vi "Read Open Thermocouple Detection.vi"(8 "error in":errorcluster, 11 "NI 9212 in":refnum<class "NI 9212.lvclass">) -> (0 "error out":errorcluster, 2 "open thermocouple detection":bool, 3 "NI 9212 out":refnum<class "NI 9212.lvclass">)   [LabVIEW 2020, in "Scan Engine Scripting.lvlib" / "NI 9212.lvclass"]
uses:
  NI 9212.lvclass
  NI 9212.lvclass/NI 9212.ctl
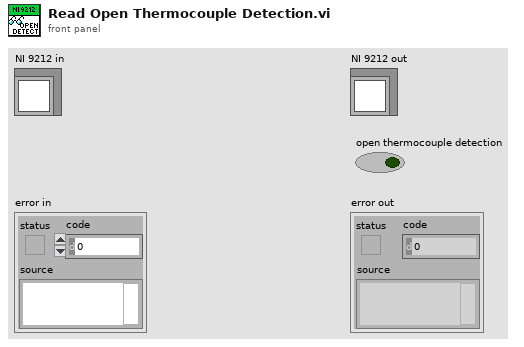
[diagram p1: front panel]
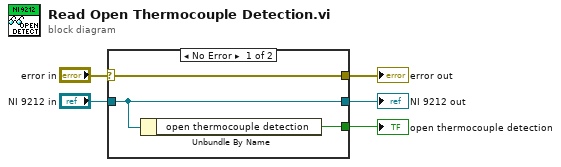
[diagram p0: block diagram]
diagram:
  n1 = case shown="No Error" "error in" {
    selector: "error in" -> [w8 w9]
    tunnel: [w8 w9] -> w4
    tunnel: [w7 w10] -> w2
    tunnel: "NI 9212 in" -> [w7 w10]
    tunnel: [w6 _] -> w1
    frame No Error {
      n2 = Unbundle By Name(w7) -> ("open thermocouple detection"=w6:bool)
    }
    frame Error {
    }
  }
  "error out" <- w4
  "NI 9212 out" <- w2
  "open thermocouple detection" <- w1
